vi "Program01 (a)].vi"() -> ()   [LabVIEW 2015]
uses:
  <vilib>/measure/NI_MABase.lvlib
panel:
  out "demodulated signal":dynamicdata(graph)=[{"t0"=timestamp(0 s since 1904-01-01), "dt"=0.0003333333333333333, "Y"=array[1000 elements], "attributes"=variant("NI_ChannelName"=variant(string "Filtered"))}]
  out "Modulated signal":waveform(dbl)(graph)={"t0"=timestamp(0 s since 1904-01-01), "dt"=0.0003333333333333333, "Y"=array[1000 elements]}
  in  "sampling info 2":cluster{"Fs":dbl, "#s":dbl}={"Fs"=3000.0, "#s"=1000.0} {"Fs" format="%.2p"}
  out "Modulating signal":waveform(dbl)(graph)={"t0"=timestamp(0 s since 1904-01-01), "dt"=0.0003333333333333333, "Y"=array[1000 elements]}
  out "Carrier Graph":waveform(dbl)(graph)={"t0"=timestamp(0 s since 1904-01-01), "dt"=0.0003333333333333333, "Y"=array[1000 elements]}
  in  "sampling info":cluster{"Fs":dbl, "#s":dbl}={"Fs"=3000.0, "#s"=1000.0} {"Fs" format="%.2p"}
  in  "signal type 2":T1(ring)
  in  "phase 2":dbl format="%.2p"
  in  "amplitude 2":dbl=1.0 format="%0.2p"
  in  "frequency 2":dbl=1000.0 format="%0.2p"
  in  "signal type":T1(ring)
  in  "phase":dbl format="%.2p"
  in  "amplitude":dbl=1.0 format="%0.2p"
  in  "frequency":dbl=10.0 format="%0.2p"
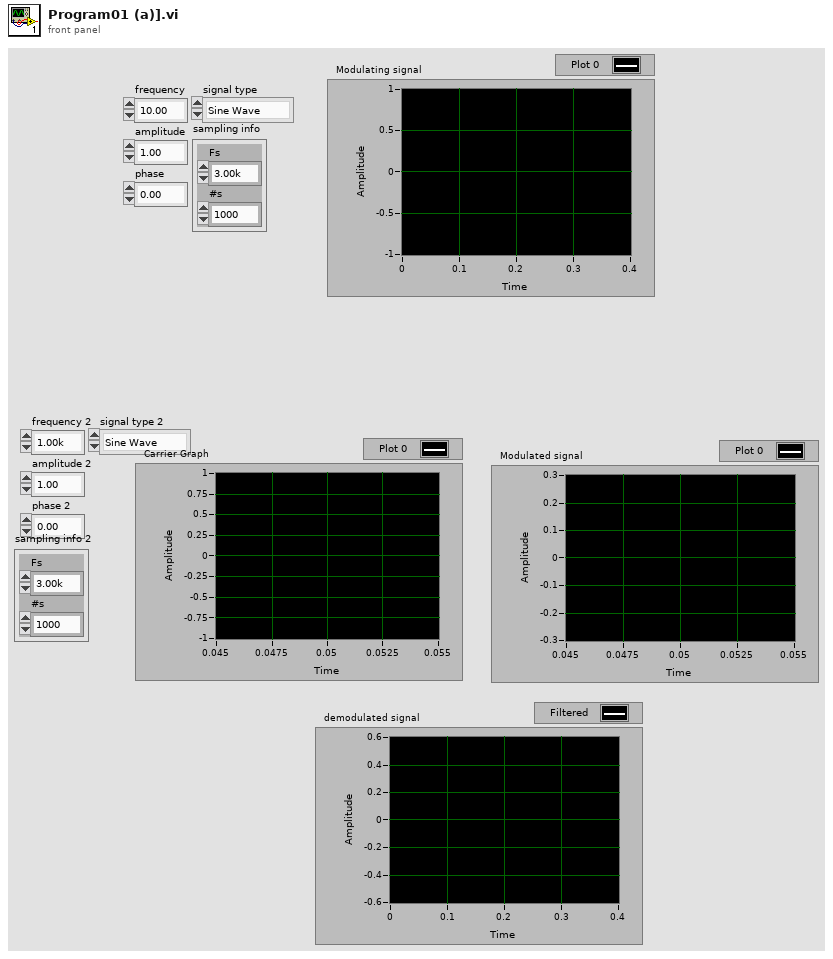
[diagram p1: front panel]
types:
  T1 = enum16{"Sine Wave", "Triangle Wave", "Square Wave", "Sawtooth Wave"}
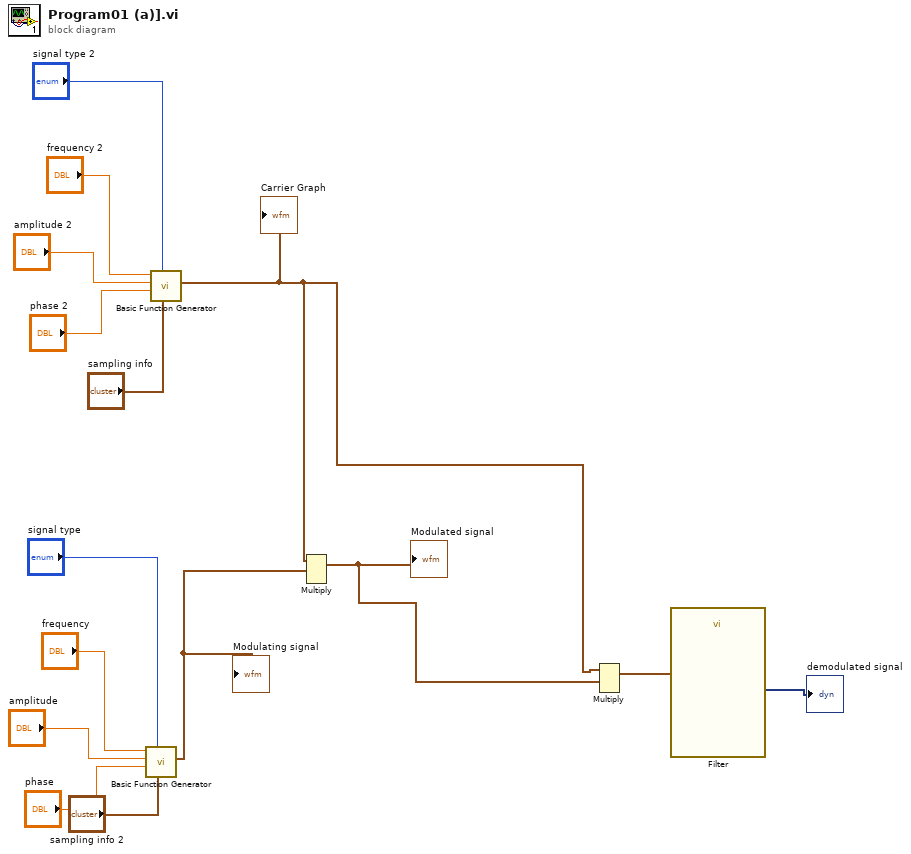
[diagram p0: block diagram]
diagram:
  n1 = call <vilib>:"Basic Function Generator.vi"("sampling info"="sampling info 2", "signal type"="signal type", "phase"="phase", "amplitude"="amplitude", "frequency"="frequency") -> ("signal out"=w6:waveform(dbl))  [unwired: 4 in, 2 out]
  "Modulating signal" <- w6
  n2 = call <vilib>:"Basic Function Generator.vi"("sampling info"="sampling info", "signal type"="signal type 2", "phase"="phase 2", "amplitude"="amplitude 2", "frequency"="frequency 2") -> ("signal out"=w4:waveform(dbl))  [unwired: 4 in, 2 out]
  "Carrier Graph" <- w4
  n3 = Multiply(1:w6, 2:w4) -> (0:w2:waveform(dbl))  [unwired: 1 in, 1 out]
  "Modulated signal" <- w2
  n4 = Multiply(1:w2, 2:w4) -> (0:w3:waveform(dbl))  [unwired: 1 in, 1 out]
  n5 = call "Filter"("Signal"=w3) -> ("Filtered Signal"=→"demodulated signal":dynamicdata)  [unwired: 9 in, 1 out]
